vi "Photometer V to C.vi"(10 "Photometer data in":T1, 11 "Volts":dbl) -> (2 "Absorbance":dbl, 3 "Concentration":dbl)   [LabVIEW 2015]
uses:
  Photometer calibration data.ctl
  <vilib>/Analysis/NI_AALPro.lvlib
panel:
  out "slope":dbl
  out "intercept":dbl
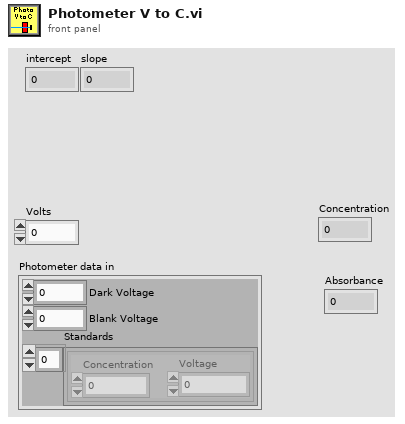
[diagram p1: front panel]
types:
  T1 = typedef "Photometer calibration data.ctl" = cluster{"Dark Voltage":dbl, "Blank Voltage":dbl, "Standards":cluster{"Concentration":dbl, "Voltage":dbl}[]}
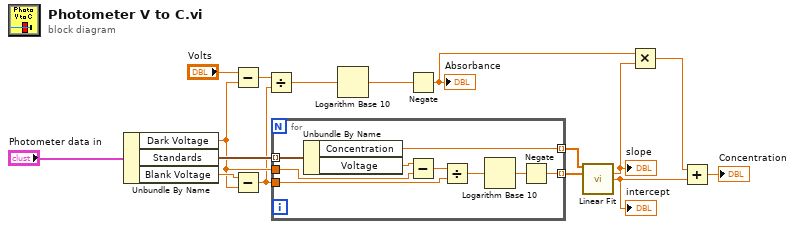
[diagram p0: block diagram]
diagram:
  n1 = Unbundle By Name("Photometer data in") -> ("Dark Voltage"=w9:dbl, "Standards"=w15:cluster{"Concentration":dbl, "Voltage":dbl}[], "Blank Voltage"=w10:dbl)
  n2 = Subtract(x="Volts", y=w9) -> (x-y=w11:dbl)
  n3 = Subtract(x=w10, y=w9) -> (x-y=w8:dbl)
  n4 = Divide(x=w11, y=w8) -> (x/y=w13:dbl)
  n5 = for {
    tunnel: w15 -> [w25] mode=indexing
    tunnel: w9 -> [w23]
    tunnel: w8 -> [w19]
    tunnel: [w18] -> w4 mode=indexing
    tunnel: [w17] -> w1 mode=indexing
    n6 = Unbundle By Name(w25) -> ("Concentration"=w17:dbl, "Voltage"=w24:dbl)
    n7 = Subtract(x=w24, y=w23) -> (x-y=w22:dbl)
    n8 = Divide(x=w22, y=w19) -> (x/y=w21:dbl)
    n9 = Logarithm Base 10(1:w21) -> (0:w20:dbl)
    n10 = Negate(x=w20) -> (-x=w18:dbl)
  }
  n11 = Logarithm Base 10(1:w13) -> (0:w14:dbl)
  n12 = Negate(x=w14) -> (-x=w2:dbl)
  "Absorbance" <- w2
  n13 = call <vilib>:"Linear Fit.vi"("Y"=w1, "X"=w4) -> ("slope"=w6:dbl, "intercept"=w5:dbl)  [unwired: 9 in, 3 out]
  "intercept" <- w5
  "slope" <- w6
  n14 = Multiply(x=w2, y=w6) -> (x*y=w7:dbl)
  n15 = Add(x=w7, y=w5) -> (x+y=→"Concentration":dbl)
